vi "Write Msg Attributes.vi"(10 "Msg Attributes":refnum<data-value>, 11 "Base Actor in":refnum<class "Base Actor.lvclass">) -> (3 "Base Actor out":refnum<class "Base Actor.lvclass">)   [LabVIEW 2020, in "jettl.lvlib" / "Base jettl Actor.lvlib" / "Base Actor.lvlib" / "Base Actor.lvclass"]
uses:
  Base Actor.lvclass
  Base Actor.lvclass/Base Actor.ctl
  Relation.ctl
  jettl.lvlib
  Teller.ctl
  Msg Attributes.ctl
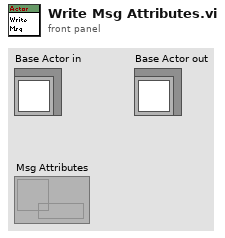
[diagram p1: front panel]
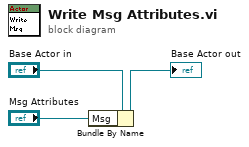
[diagram p0: block diagram]
diagram:
  n1 = Bundle By Name(cluster="Base Actor in", "Msg"="Msg Attributes") -> (→"Base Actor out":refnum<class "Base Actor.lvclass">)
